vi "create.vi"(8 "error in (no error)":errorcluster) -> (0 "error out":errorcluster, 3 "OSA200.lvclass":refnum<class "OSA200.lvclass">)   [LabVIEW 2010, in "OSA200.lvclass"]
uses:
  OSA200.lvclass
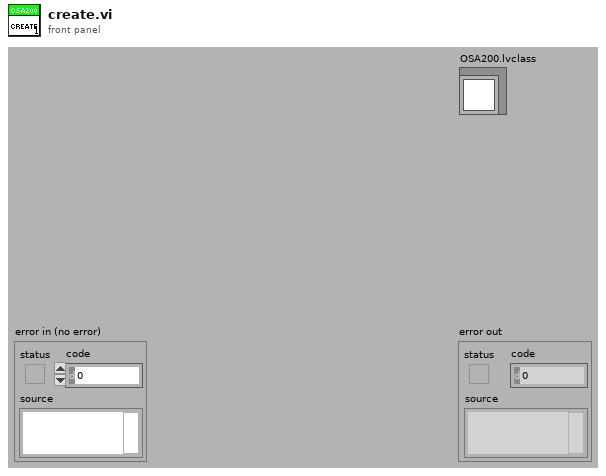
[diagram p1: front panel]
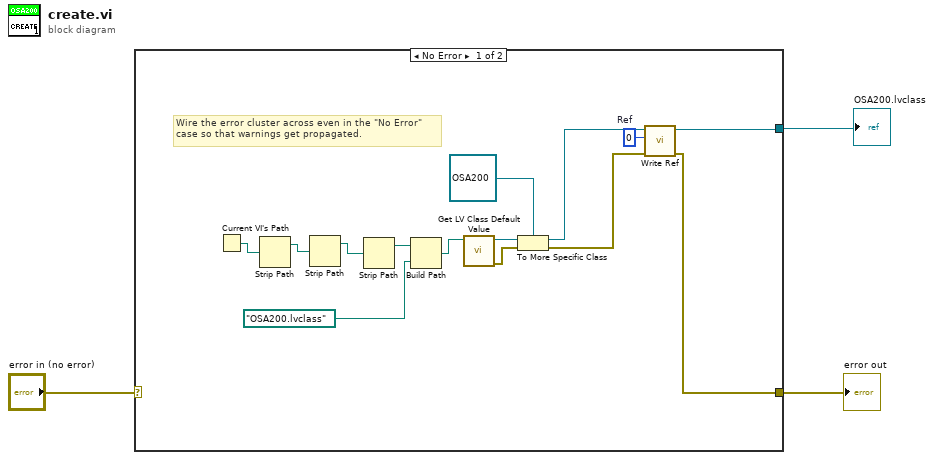
[diagram p0: block diagram]
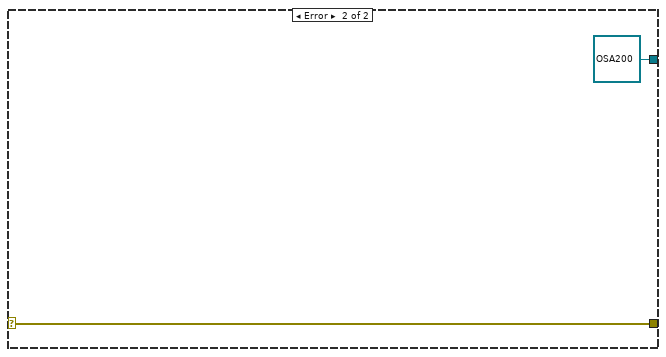
[diagram p2: hidden frame]
diagram:
  n1 = case shown="No Error" "error in (no error)" {
    selector: "error in (no error)" -> [_ w19]
    tunnel: [w4 w19] -> w2
    tunnel: [w7 refnum<class "OSA200.lvclass"> refnum ("OSA200.lvclass")] -> w1
    frame No Error {
      w6 = u32 0  # Ref
      # "Wire the error cluster across even in the \"No Error\"\ncase so that warnings get propagated."
      n2 = Current VI's Path() -> (path=w17:path)
      n3 = Strip Path(path=w17) -> (stripped path=w16:path)  [unwired: 1 out]
      n4 = Strip Path(path=w16) -> (stripped path=w15:path)  [unwired: 1 out]
      n5 = Strip Path(path=w15) -> (stripped path=w14:path)  [unwired: 1 out]
      n6 = Build Path(base path=w14, name or relative path=path "OSA200.lvclass") -> (appended path=w13:path)
      n7 = call <vilib>:"Get LV Class Default Value.vi"("class path"=w13) -> ("error out"=w10:errorcluster, "object"=w11:refnum<class>)  [unwired: 9 in]
      n8 = To More Specific Class(target class=refnum<class "OSA200.lvclass"> refnum ("OSA200.lvclass"), reference=w11, error in=w10) -> (specific class reference=w8:refnum<class "OSA200.lvclass">, error out=w5:errorcluster)
      n9 = call "Write Ref.vi"("error in (no error)"=w5, "Ref"=w6, "OSA200 in"=w8) -> ("error out"=w4:errorcluster, "OSA200 out"=w7:refnum<class "OSA200.lvclass">)  [unwired: 7 in]
    }
    frame Error {
    }
  }
  "error out" <- w2
  "OSA200.lvclass" <- w1
